vi "Async Spawn Child.vi"(6 "UID":string, 7 "Actor in":refnum<class "Actor.lvclass">, 10 "Local Layers":refnum<class "Actor.lvclass">[](array[class])) -> (0 "Error out":errorcluster, 5 "Actor out":refnum<class "Actor.lvclass">)   [LabVIEW 2025, in "jettl.lvlib"]
uses:
  jettl.lvlib
  Base Attributes/Base Attributes.lvlib
  Transport/Transport.lvclass
  Actor/Actor.lvclass
  Attributes/Attributes.lvclass
  Msg/Msg.lvclass
  Msgs.ctl
  Attributes.ctl
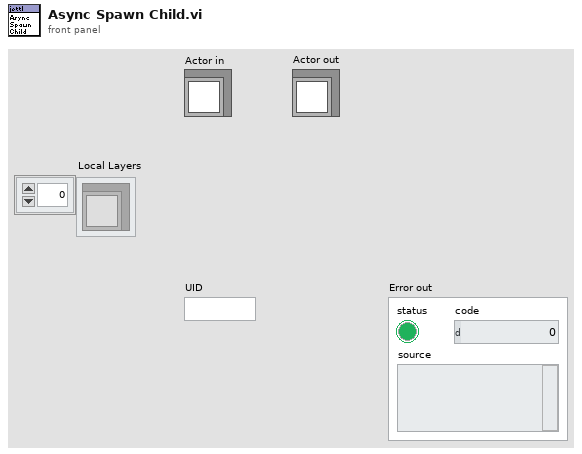
[diagram p1: front panel]
types:
  T1 = typedef "jettl.lvlib/Attributes.ctl" = cluster{"App Ref":refnum<vi>, "Persistent Actors":refnum<class "Actor.lvclass">[], "Persistent Unified Msgs":T2, "Root":bool, "UID":string, "Parent Attributes":refnum<class "Attributes.lvclass">, "Unified Msgs":T2, "VI Ref":refnum<vi>, "Transport":refnum<class "Transport.lvclass">, "Actors":refnum<class "Actor.lvclass">[]}
  T2 = typedef "jettl.lvlib/Msgs.ctl" = set{refnum<class "Msg.lvclass">}
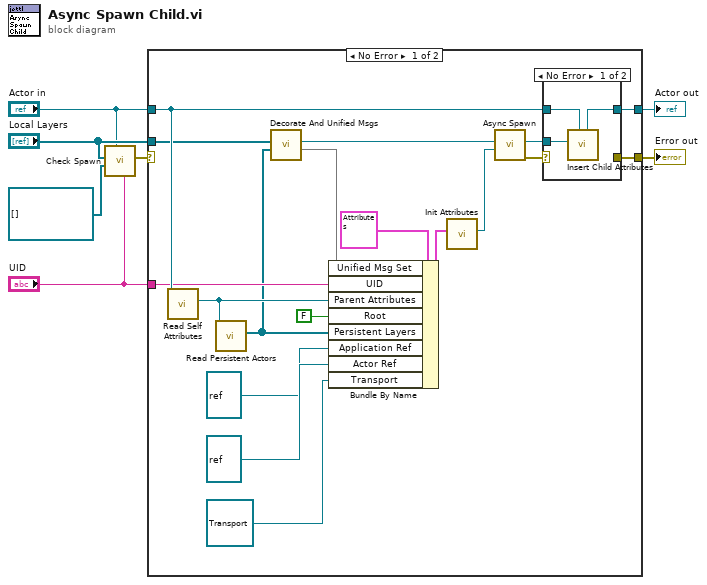
[diagram p0: block diagram]
diagram:
  n1 = call "Check Spawn.vi"("UID"="UID", "Actor in"="Actor in", "Persistent Layers"=refnum<class "Actor.lvclass">[] [], "Local Layers"="Local Layers") -> ("Error"=w5:errorcluster)  [unwired: 7 in]
  n2 = case shown="No Error" w5 {
    selector: w5 -> [_ w31]
    tunnel: "Actor in" -> [w20 w32]
    tunnel: [w23 w31] -> w7
    tunnel: [w22 w32] -> w6
    tunnel: "UID" -> [w11 _]
    tunnel: "Local Layers" -> [w16 _]
    frame No Error {
      n3 = call-dynamic "Read Self Attributes.vi"("Actor in"=w20) -> ("Self Attributes"=w10:refnum<class "Attributes.lvclass">)  [unwired: 10 in]
      n4 = call-dynamic "Read Persistent Actors.vi"("Attributes in"=w10) -> ("Persistent Actors"=w8:refnum<class "Actor.lvclass">[])  [unwired: 10 in]
      n5 = call "Decorate And Unified Msgs.vi"("Persistent Layers"=w8, "Local Layers"=w16) -> ("Unified Msg Set"=w12:T2, "Unified Actor"=w21:refnum<class "Actor.lvclass">)  [unwired: 8 in]
      n6 = Bundle By Name(cluster=T1 {"App Ref"=refnum, "Persistent Actors"=[], "Persistent Unified Msgs"={}, "Root"=FALSE, "UID"="", "Parent Attributes"=refnum, "Unified Msgs"={}, "VI Ref"=refnum, "Transport"=refnum, "Actors"=[]} ("Attributes"), "Unified Msg Set"=w12, "UID"=w11, "Parent Attributes"=w10, "Root"=FALSE, "Persistent Layers"=w8, "Application Ref"=refnum<vi> refnum, "Actor Ref"=refnum<vi> refnum, "Transport"=refnum<class "Transport.lvclass"> refnum) -> (w18:T1)
      n7 = call "Init Attributes.vi"("Attributes"=w18) -> ("Attributes"=w17:refnum<class "Attributes.lvclass">)  [unwired: 10 in]
      n8 = call "Async Spawn.vi"("Attributes"=w17, "Unified Actor"=w21) -> ("Error out"=w24:errorcluster, "Child Attributes"=w25:refnum<class "Attributes.lvclass">)  [unwired: 8 in]
      n9 = case shown="No Error" w24 {
        selector: w24 -> [_ w29]
        tunnel: w20 -> [w28 w30]
        tunnel: [w27 w30] -> w22
        tunnel: w25 -> [w26 _]
        tunnel: [_ w29] -> w23
        frame No Error {
          n10 = call "Insert Child Attributes.vi"("Actor in"=w28, "Child Attributes"=w26) -> ("Actor out"=w27:refnum<class "Actor.lvclass">)  [unwired: 9 in]
        }
        frame Error {
        }
      }
    }
    frame Error {
    }
  }
  "Actor out" <- w6
  "Error out" <- w7
